vi "close client handle.vi"(8 "error in (no error)":errorcluster, 11 "Oauth2 in":refnum<class "Oauth2.lvclass">) -> (0 "error out":errorcluster, 3 "Oauth2 out":refnum<class "Oauth2.lvclass">)   [LabVIEW 2013, in "Oauth2.lvclass"]
uses:
  Oauth2.lvclass
  Oauth2.lvclass/Oauth2.ctl
  OauthClient/OAuthClient.lvclass
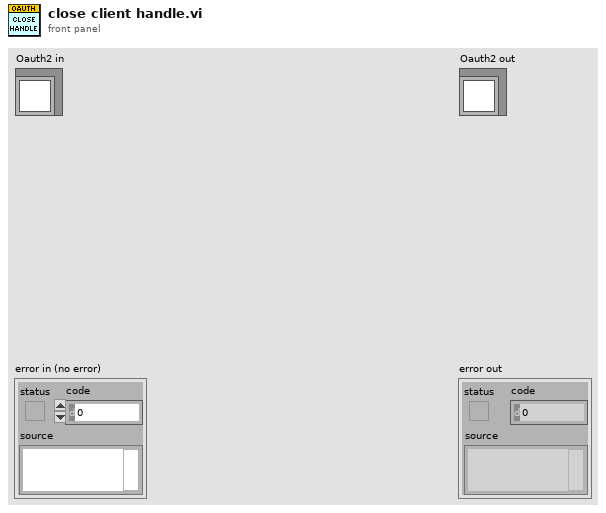
[diagram p1: front panel]
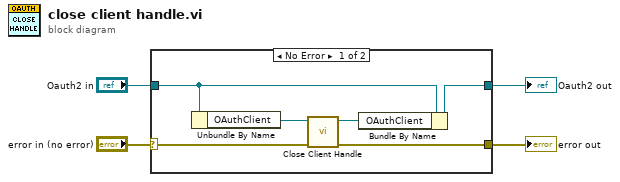
[diagram p0: block diagram]
diagram:
  n1 = case shown="No Error" "error in (no error)" {
    selector: "error in (no error)" -> [w6 w12]
    tunnel: [w5 w12] -> w3
    tunnel: [w9 w11] -> w1
    tunnel: "Oauth2 in" -> [w10 w11]
    frame No Error {
      n2 = Unbundle By Name(w10) -> ("OAuthClient"=w8:refnum<class "OAuthClient.lvclass">)
      n3 = call-dynamic "Close Client Handle.vi"("error in (no error)"=w6, "OAuthClient in"=w8) -> ("error out"=w5:errorcluster, "OAuthClient out"=w7:refnum<class "OAuthClient.lvclass">)  [unwired: 8 in]
      n4 = Bundle By Name(cluster=w10, "OAuthClient"=w7) -> (w9:refnum<class "Oauth2.lvclass">)
    }
    frame Error {
    }
  }
  "error out" <- w3
  "Oauth2 out" <- w1
